vi "Goertzel.vi"() -> ()   [LabVIEW 2014]
uses:
  <vilib>/myRIO/Express VI/Onboard IO/AI/AI Express VI.xnode
  <vilib>/myRIO/Instrument Drivers/Onboard IO/AI/vis/Read.vi
  <vilib>/myRIO/Instrument Drivers/Onboard IO/AI/AI.lvlib
  <vilib>/myRIO/Common/Instrument Driver Framework/Utilities/typedefs/Analog Scaling Constants.ctl
  <vilib>/myRIO/Common/Instrument Driver Framework/Utilities/typedefs/Analog Scaling Constants List.ctl
  <vilib>/myRIO/Common/Instrument Driver Framework/myRIO v1.0/AI/typedefs/AI Channels Enum.ctl
  <vilib>/myRIO/Common/Instrument Driver Framework/myRIO v1.0/AI/typedefs/AI Channels List.ctl
  <vilib>/myRIO/Common/Instrument Driver Framework/Utilities/typedefs/Generic FPGA Reference.ctl
  <vilib>/myRIO/Common/Instrument Driver Framework/Utilities/typedefs/myRIO v1.0 Reference.ctl
  <vilib>/myRIO/Common/Instrument Driver Framework/Utilities/typedefs/Hardware Version Enum.ctl
  <vilib>/myRIO/Common/Instrument Driver Framework/Utilities/typedefs/myRIO Generic Hardware Reference.ctl
  <vilib>/myRIO/Instrument Drivers/Onboard IO/AI/typedefs/AI Reference.ctl
  <vilib>/myRIO/Instrument Drivers/Onboard IO/AI/vis/myRIO AI Open.xnode
  <vilib>/myRIO/Common/Instrument Driver Framework/Utilities/vis/Is FPGA Ref Available.vi
  <vilib>/myRIO/Common/Instrument Driver Framework/myRIO v1.0/AI/vis/myRIO v1.1 Open AI.vi
  <vilib>/userdefined/High Color/nirio_resource_hc.ctl
  <vilib>/platform/TimedLoop/XDataNode/XDataNode.xnode
  <vilib>/Platform/TimedLoop/XDataNode/nitl_modes.ctl
  <vilib>/Platform/TimedLoop/XDataNode/XDNodeRunTimeDep.lvlib
  <vilib>/Platform/TimedLoop/XDataNode/wakeup.ctl
  <vilib>/Platform/TimedLoop/XDataNode/timing_clust.ctl
  <vilib>/myRIO/Express VI/Onboard Devices/LED/LED Express VI.xnode
  <vilib>/myRIO/Instrument Drivers/Onboard IO/DIO/vis/Write.vi
  <vilib>/myRIO/Instrument Drivers/Onboard IO/DIO/DIO.lvlib
  <vilib>/myRIO/Common/Instrument Driver Framework/myRIO v1.0/DIO/typedefs/DIO Channels Enum.ctl
  <vilib>/myRIO/Common/Instrument Driver Framework/myRIO v1.0/DIO/typedefs/DIO Channels List.ctl
  <vilib>/myRIO/Instrument Drivers/Onboard IO/DIO/typedefs/DIO Reference.ctl
  <vilib>/myRIO/Instrument Drivers/Onboard IO/DIO/vis/myRIO DIO Open.xnode
  <vilib>/myRIO/Common/Instrument Driver Framework/myRIO v1.0/DIO/vis/myRIO v1.1 Open DIO.vi
panel:
  in  "Window Length":i32=200
  out "error out":errorcluster
  in  "Stop Button":bool
  out "Input signal":dbl[](graph)=[0.017089842]
  in  "Period \n(microseconds)":i64=1000
  in  "Frequency4":dbl=941.0
  in  "Frequency3":dbl=852.0
  in  "Frequency2":dbl=770.0
  in  "Frequency1":dbl=697.0
  in  "Threshold":dbl
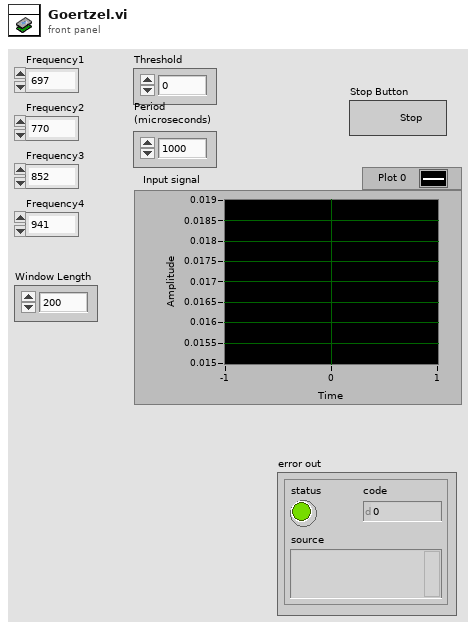
[diagram p1: front panel]
types:
  T1 = typedef "DIO.lvlib/DIO Reference.ctl" = cluster{"myRIO Reference":T2, "DIO Channels List":T6}
  T2 = typedef "myRIO Generic Hardware Reference.ctl" = cluster{"myRIO Model":T3, "myRIO Hardware Reference":T4}
  T3 = typedef "Hardware Version Enum.ctl" = enum16{"Unknown", "myRIO-1900", "myRIO-1950"}
  T4 = typedef "myRIO v1.0 Reference.ctl" = cluster{"Generic FPGA Reference":T5, "Allow multiple opens":bool}
  T5 = typedef "Generic FPGA Reference.ctl" = refnum<k20>
  T6 = typedef "DIO Channels List.ctl" = T7[]
  T7 = typedef "DIO Channels Enum.ctl" = enum16{"Not Connected", "C/DIO0", "C/DIO1", "C/DIO2", "C/DIO3", "C/DIO4", "C/DIO5", "C/DIO6", "C/DIO7", "A/DIO0", "A/DIO1", "A/DIO2", "A/DIO3", "A/DIO4", "A/DIO5", "A/DIO6", "A/DIO7", "A/DIO8", "A/DIO9", "A/DIO10", "A/DIO11", "A/DIO12", "A/DIO13", "A/DIO14", "A/DIO15", "B/DIO0", "B/DIO1", "B/DIO2", "B/DIO3", "B/DIO4", "B/DIO5", "B/DIO6", "B/DIO7", "B/DIO8", "B/DIO9", "B/DIO10", "B/DIO11", "B/DIO12", "B/DIO13", "B/DIO14", "B/DIO15", "LED0", "LED1", "LED2", "LED3", "Button0"}
  T8 = typedef "nirio_resource_hc.ctl" = tag
  T9 = typedef "AI.lvlib/AI Reference.ctl" = cluster{"myRIO Reference":T2, "AI Channels List":T10, "AI Scaling Constants List":T12}
  T10 = typedef "AI Channels List.ctl" = T11[]
  T11 = typedef "AI Channels Enum.ctl" = enum16{"Not Connected", "AudioIn/Left", "AudioIn/Right", "C/AI0", "C/AI1", "A/AI0", "A/AI1", "A/AI2", "A/AI3", "B/AI0", "B/AI1", "B/AI2", "B/AI3"}
  T12 = typedef "Analog Scaling Constants List.ctl" = T13[]
  T13 = typedef "Analog Scaling Constants.ctl" = cluster{"LSB Weight (Volts)":dbl, "Offset (Volts)":dbl, "Signed?":bool}
  T14 = typedef "XDNodeRunTimeDep.lvlib/timing_clust.ctl" = cluster{"Expected End [f-1]":u64, "Actual End [f-1]":u64, "Finished Late? [f-1]":bool, "Expected End [i-1]":u64, "Actual End [i-1]":u64, "Finished Late? [i-1]":bool, "Expected Start [i]":u64, "Actual Start [i]":u64, "Expected Start [f]":u64, "Actual Start [f]":u64, "Source Name":string, "Structure Name":string, "Period":i64, "Deadline":i64, "Offset":i64, "Start":i64, "Priority":i32, "Timeout":i32, "Mode":T15, "Wakeup Reason":T16, "Error":errorcluster, "Source Type":string, "Secondary Source Type":string, "Global End Time":u64, "Global Start Time":u64, "Frame Duration":u64, "Iteration Duration":u64, "Assigned CPU":i32, "I/O Scan Engine Mode":u32}
  T15 = typedef "XDNodeRunTimeDep.lvlib/nitl_modes.ctl" = enum32{"No Change", "Process missed periods, maintain original phase", "Discard missed periods, maintain original phase", "Process missed periods, ignore original phase", "Discard missed periods, ignore original phase"}
  T16 = typedef "XDNodeRunTimeDep.lvlib/wakeup.ctl" = enum32{"Normal", "Aborted", "Asynchronous wakeup", "Timing source error", "Timed loop error", "Timeout"}
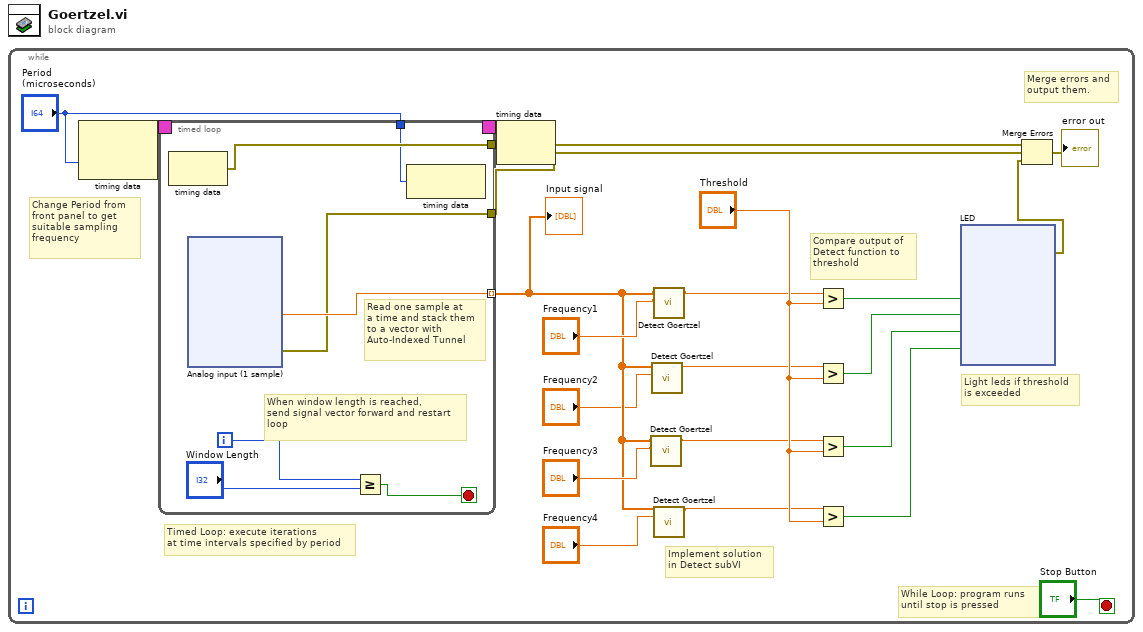
[diagram p0: block diagram]
diagram:
  n1 = while {
    stop <- "Stop Button" stop-if-true
    # "Light leds if threshold\nis exceeded"
    # "Change Period from\nfront panel to get\nsuitable sampling \nfrequency"
    # "Implement solution\nin Detect subVI"
    # "Timed Loop: execute iterations\nat time intervals specified by period"
    # "Compare output of\nDetect function to \nthreshold"
    # "Merge errors and\noutput them."
    # "While Loop: program runs\nuntil stop is pressed"
    n2 = node-c288("Period \n(microseconds)") -> (w22:T14)  [unwired: 1 in]
    n3 = timed-loop {
      timing: w22 -> [_]
      timing-out: [_] -> w21
      tunnel: [w67] -> w4 mode=indexing
      tunnel: [w66] -> _
      tunnel: [w65] -> w12
      tunnel: "Period \n(microseconds)" -> [w61]
      i -> [w64]
      stop <- w62 stop-if-true
      # "When window length is reached,\nsend signal vector forward and restart\nloop"
      # "Read one sample at \na time and stack them\nto a vector with \nAuto-Indexed Tunnel"
      n4 = node-c288() -> (w66:errorcluster)  [unwired: 1 in]
      n5 = xnode "Analog input (1 sample)"() -> ("AudioIn/Left"=w67:dbl, "error out"=w65:errorcluster)  [unwired: 1 in]
      n6 = Greater Or Equal?(x=w64, y="Window Length") -> (x >= y?=w62:bool)
      n7 = node-c288(w61) -> ()  [unwired: 1 out]
    }
    "Input signal" <- w4
    n8 = node-c288(w21) -> (w13:errorcluster)
    n9 = call "Detect Goertzel.vi"("Signal"=w4, "frequency"="Frequency3") -> ("Numeric"=w6:dbl)  [unwired: 8 in]
    n10 = call "Detect Goertzel.vi"("Signal"=w4, "frequency"="Frequency2") -> ("Numeric"=w2:dbl)  [unwired: 8 in]
    n11 = call "Detect Goertzel.vi"("Signal"=w4, "frequency"="Frequency1") -> ("Numeric"=w9:dbl)  [unwired: 8 in]
    n12 = call "Detect Goertzel.vi"("Signal"=w4, "frequency"="Frequency4") -> ("Numeric"=w7:dbl)  [unwired: 8 in]
    n13 = Greater?(x=w9, y="Threshold") -> (0:w19:bool)
    n14 = Greater?(x=w2, y="Threshold") -> (0:w18:bool)
    n15 = Greater?(x=w6, y="Threshold") -> (0:w17:bool)
    n16 = Greater?(x=w7, y="Threshold") -> (0:w16:bool)
    n17 = xnode "LED"("LED0"=w19, "LED1"=w18, "LED2"=w17, "LED3"=w16) -> ("error out"=w11:errorcluster)  [unwired: 1 in]
    n18 = Merge Errors(w13, w12, w11) -> (→"error out":errorcluster)
  }
